vi "Begin.vi"(11 "Image Size":T1=enum."160x120") -> (0 "error out":errorcluster)   [LabVIEW 2011]
doc: "Called before other user functions, this VI is expected to open initial I/O refnums, load in file data, and do all program initialization. Notice that the <B>error out</B> terminal is simply used for data flow. Wiring it to other structures or subVIs ensures that this VI runs first."
uses:
  <vilib>/Rock Robotics/WPI/Camera/WPI_CameraImageSize.ctl
  <vilib>/Rock Robotics/SystemInterfaces/DIO/FPGA_DIOPWMChannel.ctl
  <vilib>/Rock Robotics/WPI/Joystick/WPI_JoystickDeviceEnum.ctl
  <vilib>/Rock Robotics/WPI/Camera/WPI_CameraWhite Balance Values.ctl
  <vilib>/Rock Robotics/WPI/Camera/WPI_CameraExposure Values.ctl
  <vilib>/Rock Robotics/WPI/Camera/WPI_CameraFrameRate.ctl
  <vilib>/Rock Robotics/WPI/RobotDrive/WPI_RobotDriveOpen2MotorWithJaguar.vi
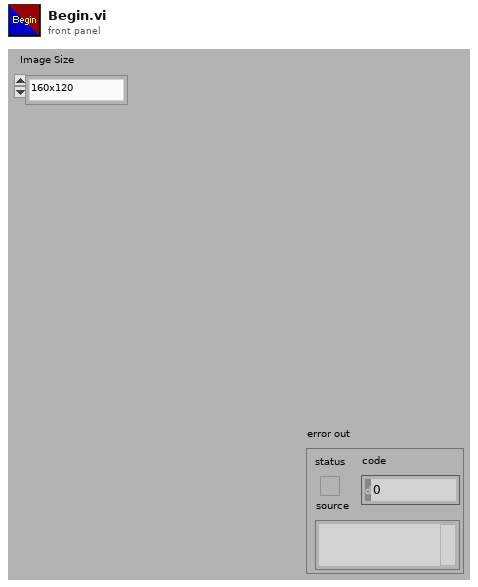
[diagram p1: front panel]
types:
  T1 = typedef "WPI_CameraImageSize.ctl" = enum16{"640x480", "320x240", "160x120"}
  T2 = typedef "WPI_JoystickDeviceEnum.ctl" = enum16{"USB 1", "USB 2", "USB 3", "USB 4", "Kinect 1", "Kinect 2"}
  T3 = typedef "WPI_CameraFrameRate.ctl" = u32
  T4 = typedef "WPI_CameraExposure Values.ctl" = enum16{"Auto", "Flicker-free 50 Hz", "Flicker-free 60 Hz", "Hold current"}
  T5 = typedef "WPI_CameraWhite Balance Values.ctl" = enum16{"Auto", "Fixed indoor", "Fixed outdoor 1", "Fixed outdoor 2", "Fixed fluorescent 1", "Fixed fluorescent 2", "Hold current"}
  T6 = typedef "FPGA_DIOPWMChannel.ctl" = enum8{"PWM 1", "PWM 2", "PWM 3", "PWM 4", "PWM 5", "PWM 6", "PWM 7", "PWM 8", "PWM 9", "PWM 10", "Invalid"}
  T7 = typedef "WPI_CameraDevRef.ctl" = cluster{"Camera Address":string, "CameraStatus":errorcluster, "Acquire Image Notifier":refnum<notifier>}
  T8 = typedef "WPI_RobotDriveDevRef.ctl" = cluster{"DevStatus":errorcluster, "Motors[]":T9[], "Square Inputs":bool, "Max Output":dbl, "Isochronous":bool}
  T9 = typedef "WPI_MotorControlDeviceRef.ctl" = cluster{"DeviceStatus":errorcluster, "Type":enum16{"PWM", "CAN"}, "PWM":cluster{"Digital Module":T10, "PWM Channel":T6, "DeadBand":T11}, "CAN":cluster{"Device Number":u8, "Control Mode":T12, "Semaphore":T13, "Max Vout":dbl}, "Invert":bool, "TransformRef":T14, "InvTransformRef":T14}
  T10 = typedef "FPGA_TypedefDigitalModule.ctl" = enum16{"Digital Module 1", "Digital Module 2"}
  T11 = typedef "WPI_PWMDeadband.ctl" = cluster{"Name":string, "maxPositivePwm":i32, "minPositivePwm":i32, "centerPwm":i32, "maxNegativePwm":i32, "minNegativePwm":i32, "angularRange":u16}
  T12 = typedef "WPI_CANJaguar_ControlMode.ctl" = enum8{"Percent VBus", "Current", "Speed", "Position", "Voltage"}
  T13 = typedef "Semaphore RefNum" = refnum<k1>
  T14 = typedef "WPI_PWMTransform_ConPane.ctl" = refnum<vi>
  T15 = typedef "WPI_JoystickDevRef.ctl" = cluster{"Device":T2}
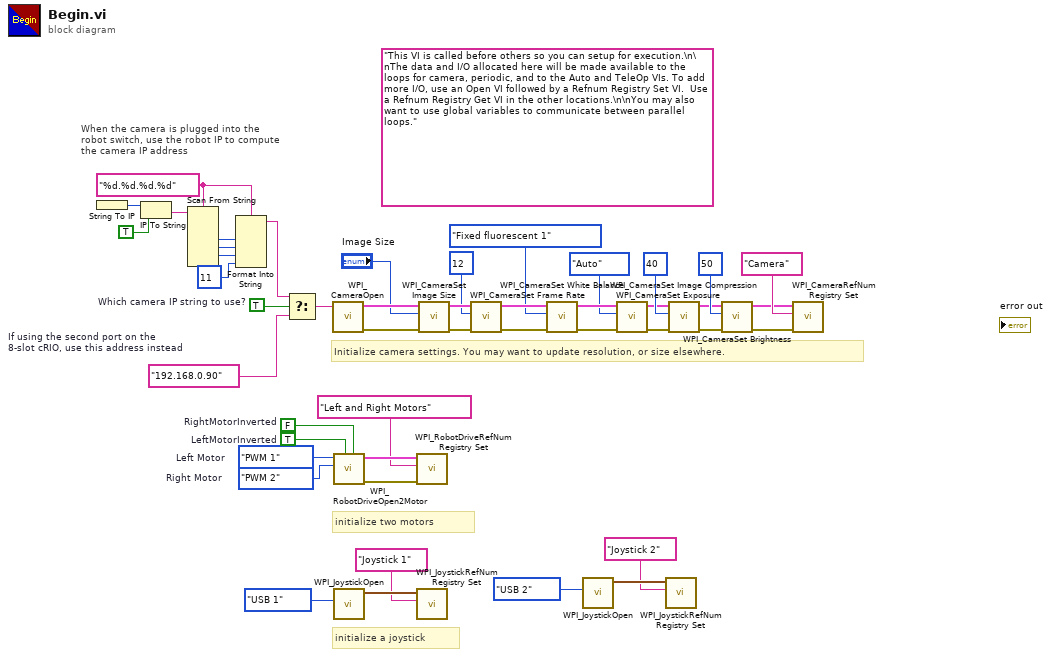
[diagram p0: block diagram]
diagram:
  w4 = TRUE  # Which camera IP string to use?
  w8 = "%d.%d.%d.%d" ("format string")
  (unwired) "This VI is called before others so you can setup for execution.\n\nThe data and I/O allocated here will be made available to the loops for camera, periodic, and to the Auto and TeleOp VIs. To add more I/O, use an Open VI followed by a Refnum Registry Set VI.  Use a Refnum Registry Get VI in the other locations.\n\nYou may also want to use global variables to communicate between parallel loops."
  w20 = FPGA_DIOPWMChannel."PWM 2"  # Right Motor
  w21 = FPGA_DIOPWMChannel."PWM 1"  # Left Motor
  w5 = "192.168.0.90"  # If using the second port on the 8-slot cRIO, use this address instead
  w45 = TRUE  # LeftMotorInverted
  w46 = FALSE  # RightMotorInverted
  # "When the camera is plugged into the\nrobot switch, use the robot IP to compute\nthe camera IP address"
  # "initialize a joystick"
  # "initialize two motors"
  # "Initialize camera settings. You may want to update resolution, or size elsewhere."
  n1 = String To IP() -> (0:w15:u32)  [unwired: 1 in]
  n2 = IP To String(1:TRUE ("dot notation? (F)"), 2:w15) -> (0:w13:string)
  n3 = Scan From String(format string=w8, input string=w13) -> (output 1=w12:i32, output 2=w11:i32, output 3=w10:i32)  [unwired: 7 in, 3 out]
  n4 = Format Into String(format string=w8, w12, w11, w10, 11 ("Compression")) -> (resulting string=w6:string)  [unwired: 2 in, 1 out]
  n5 = Select(t=w6, s=w4, f=w5) -> (s? t:f=w7:string)
  n6 = call <vilib>:"WPI_CameraOpen.vi"("Camera Address"=w7) -> ("error out"=w30:errorcluster, "CameraDevRef"=w31:T7)  [unwired: 1 in, 8 out]
  n7 = call-poly <vilib>:"WPI_RobotDriveOpen2Motor.vi"("Right Motor Inverted"=w46, "Left Motor Inverted"=w45, "Right Motor"=w20, "Left Motor"=w21) -> ("error out"=w39:errorcluster, "RobotDriveDevRef"=w43:T8)  [unwired: 1 in, 5 out]
  n8 = call <vilib>:"WPI_JoystickOpen.vi"("JoystickDevice"=WPI_JoystickDeviceEnum."USB 1") -> ("JoystickDevRef"=w41:T15)  [unwired: 10 out]
  n9 = call <vilib>:"WPI_RobotDriveRefNum Registry Set.vi"("error in (no error)"=w39, "refnum name"="Left and Right Motors", "RobotDriveDevRef"=w43) -> ()  [unwired: 9 out]
  n10 = call <vilib>:"WPI_JoystickRefNum Registry Set.vi"("refnum name"="Joystick 1", "JoystickDevRef"=w41) -> ()  [unwired: 1 in, 9 out]
  n11 = call <vilib>:"WPI_CameraSet Image Size.vi"("error in (no error)"=w30, "Image Size"="Image Size", "CameraDevRef"=w31) -> ("error out"=w29:errorcluster, "CameraDevRef Out"=w32:T7)  [unwired: 7 out]
  n12 = call <vilib>:"WPI_CameraSet Frame Rate.vi"("error in (no error)"=w29, "Frame Rate (fps)"=T3 12, "CameraDevRef"=w32) -> ("error out"=w28:errorcluster, "CameraDevRef Out"=w34:T7)  [unwired: 7 out]
  n13 = call <vilib>:"WPI_CameraSet White Balance.vi"("error in (no error)"=w28, "White Balance"=WPI_CameraWhite_Balance_Values."Fixed fluorescent 1", "CameraDevRef"=w34) -> ("error out"=w27:errorcluster, "CameraDevRef Out"=w33:T7)  [unwired: 7 out]
  n14 = call <vilib>:"WPI_JoystickOpen.vi"("JoystickDevice"=WPI_JoystickDeviceEnum."USB 2") -> ("JoystickDevRef"=w3:T15)  [unwired: 10 out]
  n15 = call <vilib>:"WPI_CameraSet Exposure.vi"("error in (no error)"=w27, "Exposure"=WPI_CameraExposure_Values."Auto", "CameraDevRef"=w33) -> ("error out"=w26:errorcluster, "CameraDevRef Out"=w36:T7)  [unwired: 7 out]
  n16 = call <vilib>:"WPI_JoystickRefNum Registry Set.vi"("refnum name"="Joystick 2", "JoystickDevRef"=w3) -> ()  [unwired: 1 in, 9 out]
  n17 = call <vilib>:"WPI_CameraSet Image Compression.vi"("error in (no error)"=w26, "Compression"=40, "CameraDevRef"=w36) -> ("error out"=w25:errorcluster, "CameraDevRef Out"=w35:T7)  [unwired: 7 out]
  n18 = call <vilib>:"WPI_CameraSet Brightness.vi"("error in (no error)"=w25, "Brightness"=50, "CameraDevRef"=w35) -> ("error out"=w23:errorcluster, "CameraDevRef Out"=w24:T7)  [unwired: 7 out]
  n19 = call <vilib>:"WPI_CameraRefNum Registry Set.vi"("error in (no error)"=w23, "refnum name"="Camera", "CameraDevRef"=w24) -> ()  [unwired: 9 out]
